vi "量程参数设置.vi"(10 "自动测试量程配置":T4, 11 "质控参数设置":T2) -> (1 "checkout":bool, 2 "CODMn自动测试量程配置 2":T4, 3 "输出簇":T1)   [LabVIEW 2016, in "斯坦道CODMn新电路板.lvlib"]
uses:
  <vilib>/Utility/miscctls.llb/LVPointTypeDef.ctl
panel:
  in  "codmn标准液标准浓度":dbl
  in  "codmn跨度标准液浓度":dbl
  in  "codmn零点标准液浓度":dbl
  in  "codmn跨度值":dbl
  in  "取消":bool
  in  "确定":bool
  # "量程、质控参数设置"
  # "质控上传平台参数设置"
  # "跨度值"
  # "mg/L"
  # "零点核查标准液浓度"
  # "mg/L"
  # "跨度核查标准液浓度"
  # "mg/L"
  # "标样核查标准液浓度"
  # "mg/L"
  # "质控参数设置"
  # "监测参数"
  # "codmn"
  # "跨度值"
  # "零点核查标准液浓度"
  # "跨度核查标准液浓度"
  # "标样核查标准液浓度"
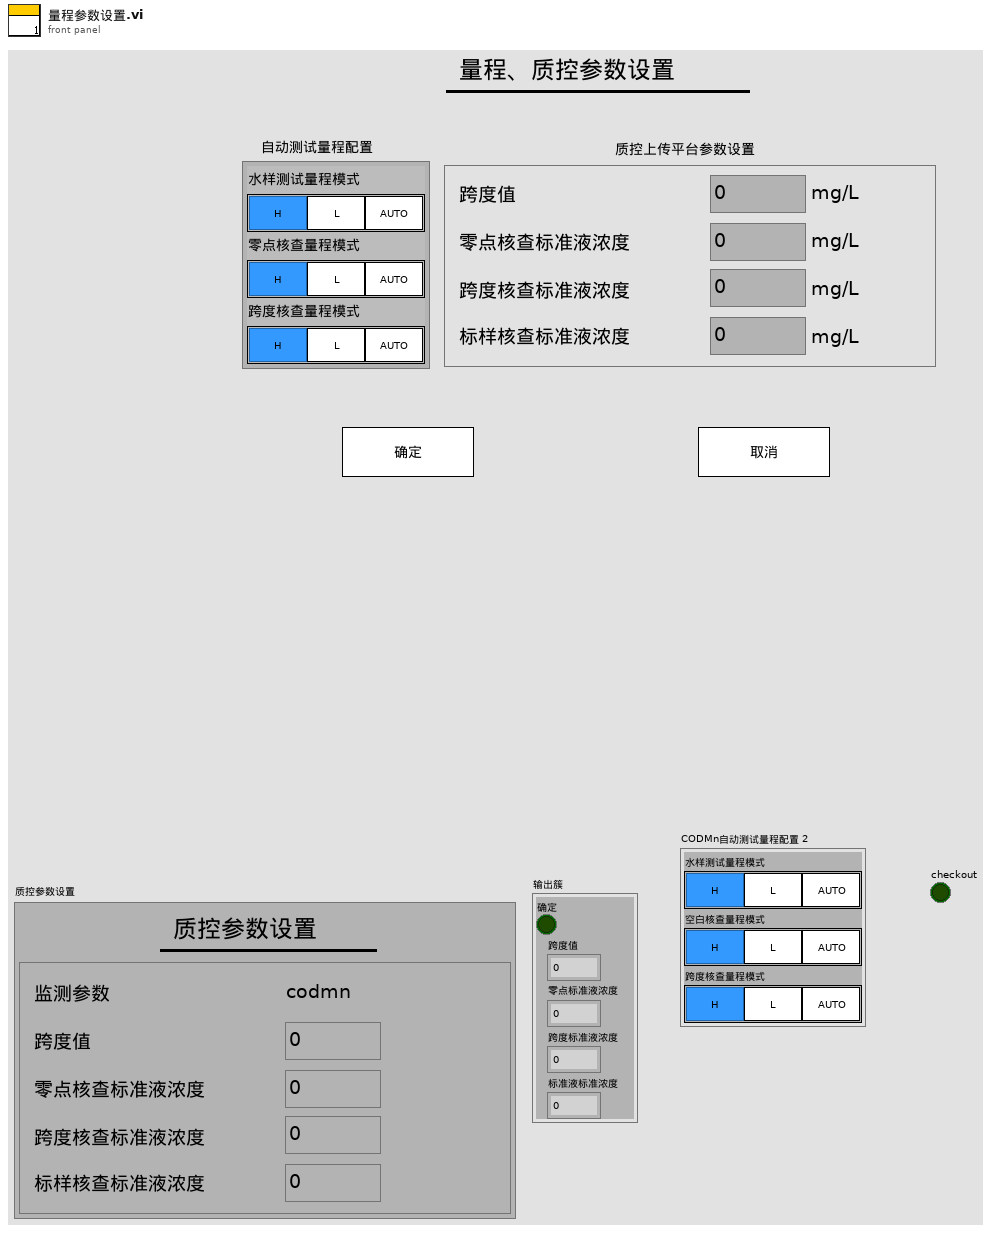
[diagram p1: front panel]
types:
  T1 = cluster{"确定":bool, "跨度值":dbl, "零点标准液浓度":dbl, "跨度标准液浓度":dbl, "标准液标准浓度":dbl}
  T2 = cluster{"总磷跨度值":dbl, "总磷零点标准液浓度":dbl, "总磷跨度标准液浓度":dbl, "总磷标准液标准浓度":dbl}
  T3 = typedef "量程选择控件.ctl" = enum32{"H", "L", "AUTO"}
  T4 = cluster{"水样测试量程模式":T3, "空白核查量程模式":T3, "跨度核查量程模式":T3}
  T5 = typedef "LVPointTypeDef.ctl" = cluster{"Horizontal":i16, "Vertical":i16}
  T6 = cluster{"确定":bool, "codmn跨度值":dbl, "codmn零点标准液浓度":dbl, "codmn跨度标准液浓度":dbl, "codmn标准液标准浓度":dbl}
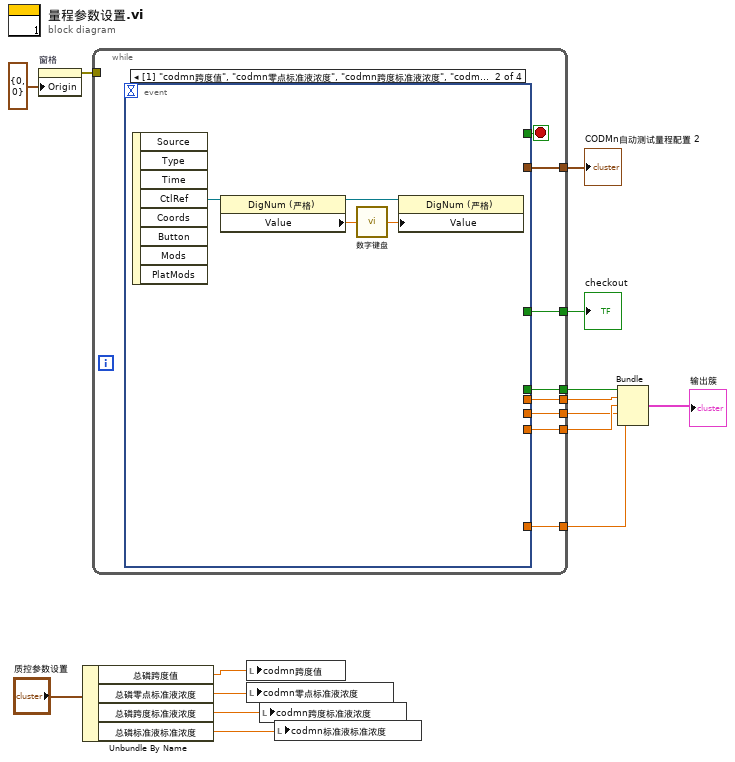
[diagram p0: block diagram]
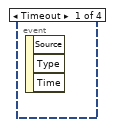
[diagram p2: hidden frame]
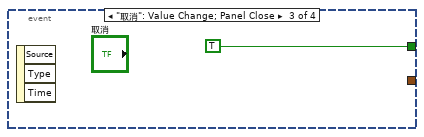
[diagram p3: hidden frame]
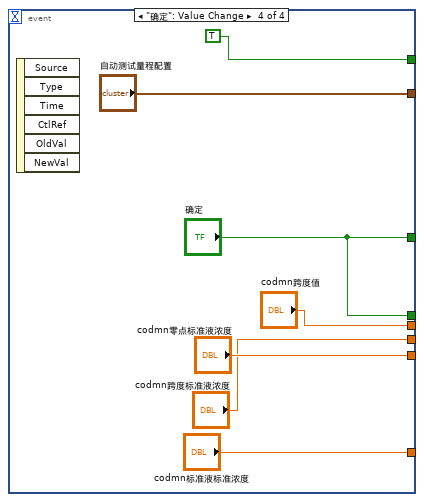
[diagram p4: hidden frame]
diagram:
  n1 = property on="窗格" class="Pane"("Origin"=T5 {"Horizontal"=0, "Vertical"=0} ("原点")) -> (error out=w14:errorcluster)  [unwired: 2 in, 1 out]
  n2 = Unbundle By Name("质控参数设置") -> ("总磷跨度值"=w10:dbl, "总磷零点标准液浓度"=w9:dbl, "总磷跨度标准液浓度"=w8:dbl, "总磷标准液标准浓度"=w7:dbl)
  n3 = while {
    tunnel: w14 -> [_]
    tunnel: [w22] -> w13
    tunnel: [w21] -> w12
    tunnel: [w20] -> w6
    tunnel: [w19] -> w5
    tunnel: [w18] -> w4
    tunnel: [w17] -> w3
    tunnel: [w16] -> w2
    stop <- w23 stop-if-true
    n4 = event shown="[1] \"codmn跨度值\", \"codmn零点标准液浓度\", \"codmn跨度标准液浓度\", \"codmn标准液标准浓度\": 鼠标按下" {
      selector: _ -> [_ _ _ _]
      dyn-events: _ -> [_ _ _ _]
      timeout: _ -> [_ _ _ _]
      tunnel: [_ _ TRUE TRUE] -> w23
      tunnel: [_ _ _ "确定"] -> w22
      tunnel: [_ _ _ "自动测试量程配置"] -> w21
      tunnel: [_ _ _ "确定"] -> w20
      tunnel: [_ _ _ "codmn跨度值"] -> w19
      tunnel: [_ _ _ "codmn零点标准液浓度"] -> w18
      tunnel: [_ _ _ "codmn跨度标准液浓度"] -> w17
      tunnel: [_ _ _ "codmn标准液标准浓度"] -> w16
      event Timeout {
        n5 = event-data() -> ()  [unwired: 1 in, 3 out]
      }
      event "codmn跨度值", "codmn零点标准液浓度", "codmn跨度标准液浓度", "codmn标准液标准浓度": Mouse Down {
        n6 = event-data() -> ("CtlRef"=w24:refnum<vi>)  [unwired: 1 in, 7 out]
        n7 = property class="DigNum (严格)"(reference=w24) -> (reference out=w27:refnum<vi>, "Value"=w26:dbl)  [unwired: 1 in, 1 out]
        n8 = call "数字键盘.vi"("OldNumber"=w26) -> ("NewNumber"=w25:dbl)
        n9 = property class="DigNum (严格)"(reference=w27, "Value"=w25) -> ()  [unwired: 1 in, 2 out]
      }
      event "取消": Value Change; Panel Close {
        n10 = event-data() -> ()  [unwired: 1 in, 3 out]
      }
      event "确定": Value Change {
        n11 = event-data() -> ()  [unwired: 1 in, 6 out]
      }
    }
  }
  "checkout" <- w13
  "CODMn自动测试量程配置 2" <- w12
  n12 = local write "codmn跨度值"(w10) -> ()
  n13 = local write "codmn零点标准液浓度"(w9) -> ()
  n14 = local write "codmn跨度标准液浓度"(w8) -> ()
  n15 = local write "codmn标准液标准浓度"(w7) -> ()
  n16 = Bundle("确定"=w6, "codmn跨度值"=w5, "codmn零点标准液浓度"=w4, "codmn跨度标准液浓度"=w3, "codmn标准液标准浓度"=w2) -> (→"输出簇":T6)  [unwired: 1 in]
